vi "RotateWall.vi"(8 "Move amount in":dbl, 9 "Acceleration (deg2/s)":dbl, 10 "Speed (deg/s)":dbl, 11 "Physical step size (deg/step)":dbl) -> (0 "StepTimes":cluster{dbl, "y":dbl}[](array[cluster]), 3 "ActualMovement":dbl)   [LabVIEW 2013]
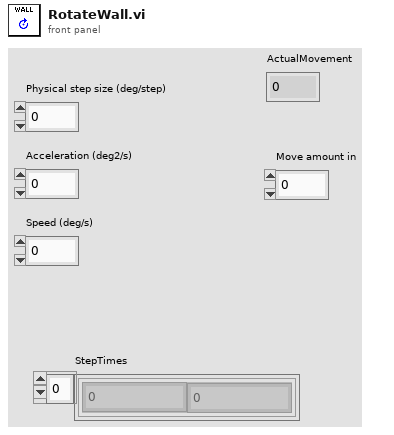
[diagram p1: front panel]
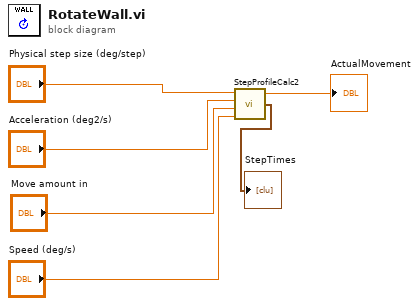
[diagram p0: block diagram]
diagram:
  n1 = call "StepProfileCalc2.vi"("Max speed"="Speed (deg/s)", "Move amount"="Move amount in", "Acceleration"="Acceleration (deg2/s)", "Step size"="Physical step size (deg/step)") -> ("StepTimes"=→"StepTimes":cluster{dbl, "y":dbl}[], "ActualMovement"=→"ActualMovement":dbl)  [unwired: 1 in]
